vi "Quick Start.vi"() -> ()   [LabVIEW 2020]
uses:
  Source/LV Logging.lvlib
  Source/Type Defs/Debug Level.ctl
  <vilib>/Utility/sysdir.llb/System Directory Type.ctl
panel:
  in  "error in (no error)":errorcluster
  out "error out":errorcluster
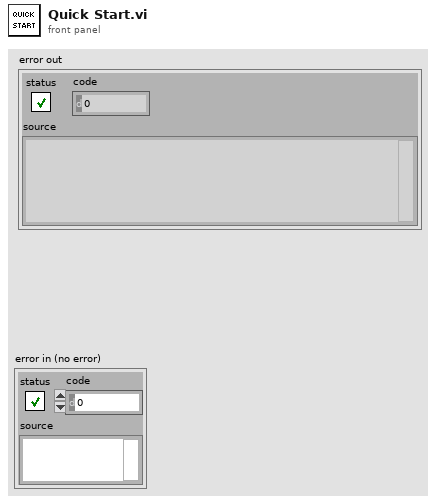
[diagram p1: front panel]
types:
  T1 = typedef "System Directory Type.ctl" = i32
  T2 = typedef "LV Logging.lvlib/Debug Level.ctl" = enum16{"DEBUG", "INFO", "WARN", "ERROR", "FATAL"}
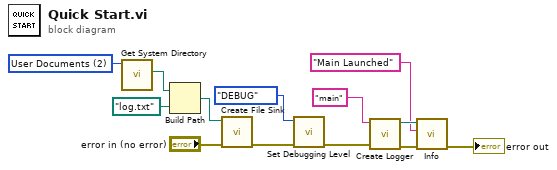
[diagram p0: block diagram]
diagram:
  w2 = T1 2 items=["User Home"=0, "User Desktop"=1, "User Documents"=2, "User Application Data"=3, "User Preferences"=4, "User Temporary"=5, "Public Documents"=6, "Public Application Data"=7, "Public Preferences"=8, "Public Cache"=13, "System Core Libraries"=9, "System Installed Libraries"=10, "Application Files"=11, "Boot Volume Root"=12] ("system directory type")
  n1 = call <vilib>:"Get System Directory.vi"("system directory type"=w2) -> ("system directory"=w1:path)  [unwired: 10 in]
  n2 = Build Path(base path=w1, name or relative path=path "log.txt") -> (appended path=w3:path)
  n3 = call "Create File Sink.vi"("error in (no error)"="error in (no error)", "Path"=w3) -> ("error out"=w12:errorcluster)  [unwired: 9 in]
  n4 = call "Set Debugging Level.vi"("error in (no error)"=w12, "Debug Level in"=Debug_Level."DEBUG" ("Debug Level")) -> ("error out"=w10:errorcluster)  [unwired: 9 in]
  n5 = call "Create Logger.vi"("error in (no error)"=w10, "Name"="main") -> ("error out"=w9:errorcluster, "Logger out"=w8:refnum<class "Logger.lvclass">)  [unwired: 8 in]
  n6 = call "Info.vi"("error in (no error)"=w9, "Log Text"="Main Launched", "Logger in"=w8) -> ("error out"=→"error out":errorcluster)  [unwired: 7 in, 1 out]
